vi "DetectCollisionImproved.vi"(0 "ball":dbl[](array[numeric]), 4 "Goal":dbl[](array[numeric]), 5 "our_robots":T1[](array[typedef]), 6 "Initial State":dbl[](array[numeric]), 7 "enemy_robots":T1[](array[typedef]), 8 "Is not first robot?":bool, 9 "element being analyzed":dbl[](array[numeric]), 10 "element already in path":dbl[](array[numeric]), 11 "Robot in":T1) -> (2 "Is there colision?":bool)   [LabVIEW 2017]
uses:
  Core/AI Robot.ctl
  Intel/Functions Enum.ctl
  Intel/AttackerStates.ctl
  PathDests.ctl
  PathDest.ctl
  <vilib>/Analysis/_algsub.llb/Real Vector Norm.vi
  <vilib>/Analysis/baseanly.llb/Real Dot Product.vi
  <vilib>/Analysis/NI_AALBase.lvlib
  <vilib>/Analysis/NI_AALPro.lvlib
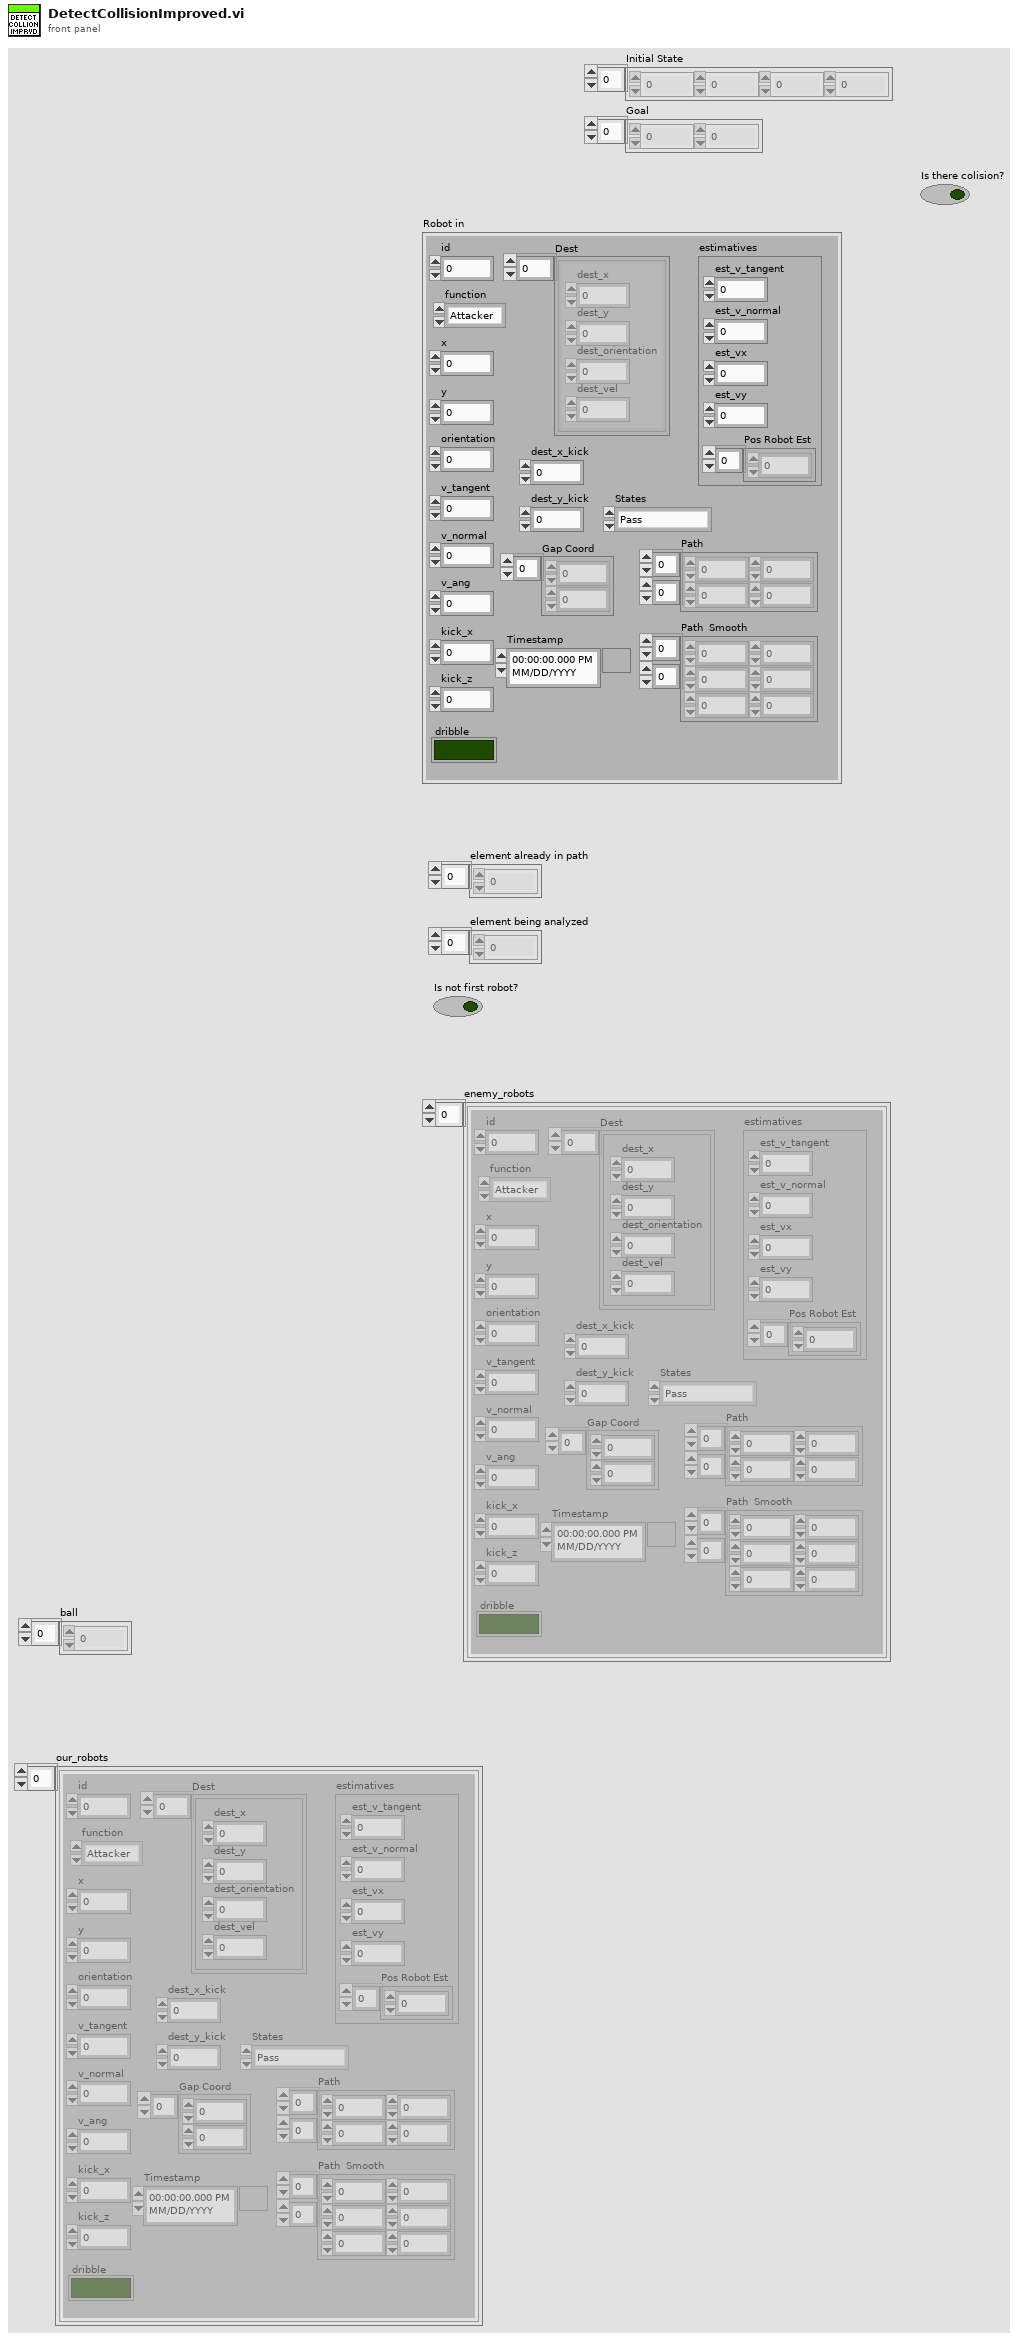
[diagram p1: front panel]
types:
  T1 = typedef "AI Robot.ctl" = cluster{"id":u32, "function":T2, "x":dbl, "y":dbl, "orientation":dbl, "v_tangent":dbl, "v_normal":dbl, "v_ang":dbl, "kick_x":dbl, "kick_z":dbl, "dribble":bool, "Timestamp":timestamp, "estimatives":cluster{"est_v_tangent":dbl, "est_v_normal":dbl, "est_vx":dbl, "est_vy":dbl, "Pos Robot Est":dbl[]}, "dest_x_kick":dbl, "dest_y_kick":dbl, "Gap Coord":dbl[], "States":T3, "Path ":dbl[][], "Path  Smooth":dbl[][], "Dest":T4}
  T2 = typedef "Functions Enum.ctl" = enum16{"Attacker", "Goalie", "Defender", "Striker", "Goto 0", "Dummy", "Kicker", "ZigZag"}
  T3 = typedef "AttackerStates.ctl" = enum16{"Pass", "GoToTangent", "BallGetting", "GoToKick", ""}
  T4 = typedef "PathDests.ctl" = T5[]
  T5 = typedef "PathDest.ctl" = cluster{"dest_x":dbl, "dest_y":dbl, "dest_orientation":dbl, "dest_vel":dbl}
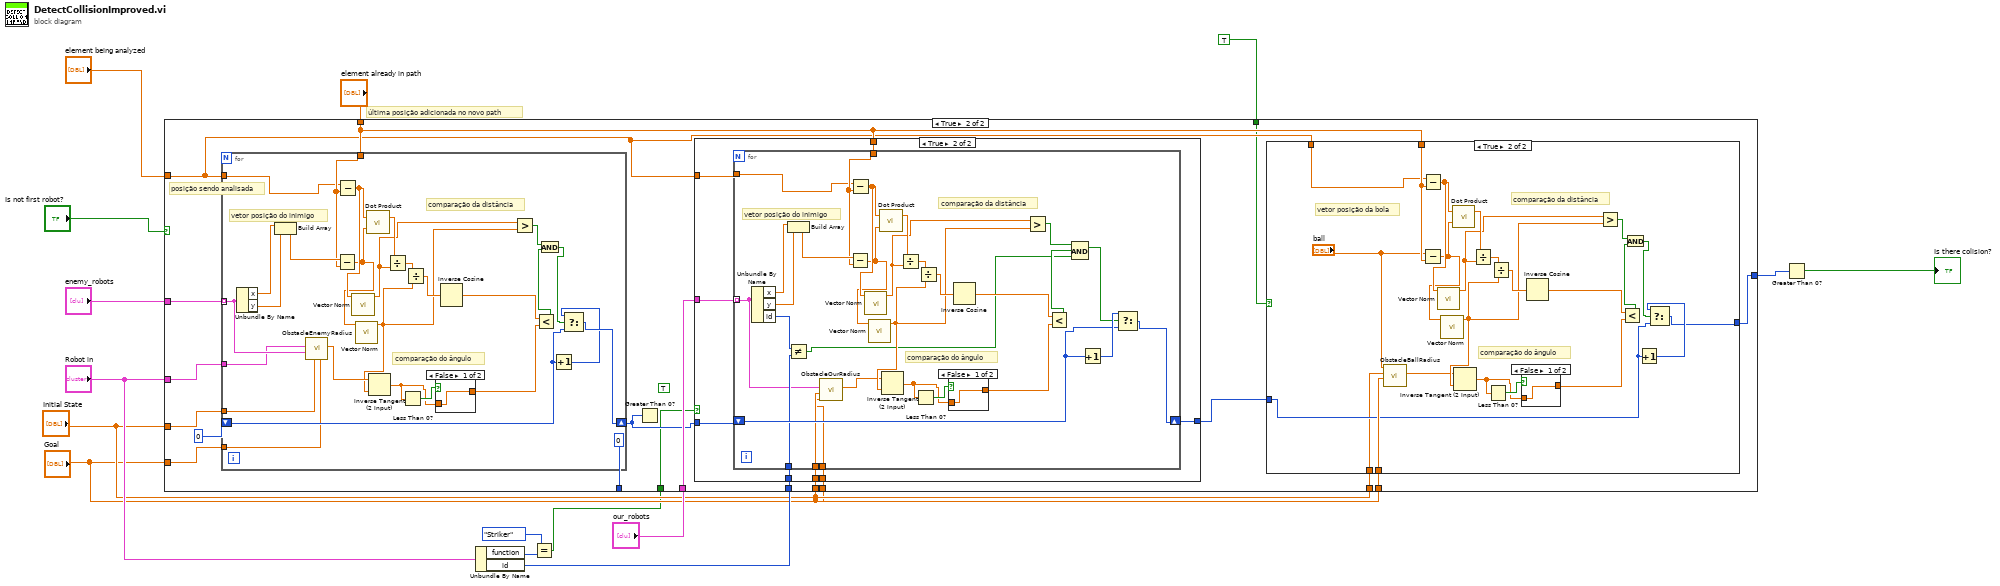
[diagram p0: block diagram]
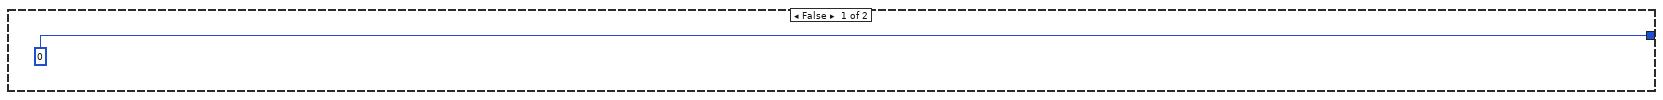
[diagram p2: hidden frame]
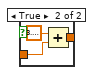
[diagram p4: hidden frame]
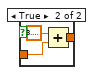
[diagram p6: hidden frame]
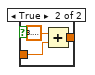
[diagram p7: hidden frame]
diagram:
  # "última posição adicionada no novo path"
  n1 = Unbundle By Name("Robot in") -> ("function"=w3:T2, "id"=w7:u32)
  n2 = Equal?(x=Functions_Enum."Striker", y=w3) -> (x = y?=w1:bool)
  n3 = case shown="True" "Is not first robot?" {
    tunnel: "enemy_robots" -> [_ w35]
    tunnel: "element being analyzed" -> [_ w23]
    tunnel: "element already in path" -> [_ w24]
    tunnel: [0 w20] -> w15
    tunnel: "Robot in" -> [_ w33]
    tunnel: "Initial State" -> [_ w32]
    tunnel: "Goal" -> [_ w31]
    tunnel: 0 -> [_ _]
    tunnel: "our_robots" -> [_ w30]
    tunnel: w7 -> [_ w29]
    tunnel: "Initial State" -> [_ w27]
    tunnel: "Goal" -> [_ w26]
    tunnel: "Initial State" -> [_ w22]
    tunnel: "Goal" -> [_ w21]
    tunnel: TRUE -> [_ w19]
    tunnel: w1 -> [_ w18]
    frame False {
    }
    frame True {
      (unwired) TRUE
      # "posição sendo analisada"
      n4 = for {
        tunnel: w35 -> [w111] mode=indexing
        shift-right: [w121] -> w28
        shift-left: 0 -> [w119]
        tunnel: w23 -> [w128]
        tunnel: w24 -> [w129]
        tunnel: w33 -> [w110]
        tunnel: w32 -> [w109]
        tunnel: w31 -> [w108]
        # "comparação do ângulo"
        # "comparação da distância"
        # "vetor posição do inimigo"
        n5 = Unbundle By Name(w111) -> ("x"=w132:dbl, "y"=w131:dbl)
        n6 = Build Array(w132, w131) -> (w130:dbl[])
        n7 = call "ObstacleEnemyRadius.vi"("Goal"=w108, "Initial State"=w109, "Robot enemy"=w111, "Robot in"=w110) -> ("obstacle enemy radius"=w107:dbl)  [unwired: 7 in]
        n8 = Subtract(x=w130, y=w129) -> (x-y=w122:dbl[])
        n9 = Subtract(x=w128, y=w129) -> (x-y=w126:dbl[])
        n10 = call-poly <vilib>:"Vector Norm.vi"("Input Vector"=w126) -> ("norm"=w118:dbl)  [unwired: 9 in, 1 out]
        n11 = call-poly <vilib>:"Vector Norm.vi"("Input Vector"=w122) -> ("norm"=w106:dbl)  [unwired: 9 in, 1 out]
        n12 = call-poly <vilib>:"Dot Product.vi"("Y Vector"=w122, "X Vector"=w126) -> ("X * Y"=w127:dbl)  [unwired: 1 out]
        n13 = Inverse Tangent (2 Input)(1:w106, 2:w107) -> (0:w113:dbl)
        n14 = Divide(x=w127, y=w118) -> (x/y=w125:dbl)
        n15 = Less Than 0?(x=w113) -> (x < 0?=w114:bool)
        n16 = Divide(x=w125, y=w106) -> (x/y=w124:dbl)
        n17 = case shown="False" w114 {
          tunnel: w113 -> [w133 w135]
          tunnel: [w133 w134] -> w112
          frame False {
          }
          frame True {
            n18 = Add(x=3.141592653589793, y=w135) -> (x+y=w134:dbl)
          }
        }
        n19 = Inverse Cosine(1:w124) -> (0:w123:dbl)
        n20 = Greater?(x=w118, y=w106) -> (0:w117:bool)
        n21 = Less?(x=w123, y=w112) -> (x < y?=w116:bool)
        n22 = And(x=w117, y=w116) -> (x .and. y?=w115:bool)
        n23 = Increment(x=w119) -> (x+1=w120:i32)
        n24 = Select(t=w120, s=w115, f=w119) -> (s? t:f=w121:i32)
      }
      n25 = Greater Than 0?(x=w28) -> ()  [unwired: 1 out]
      n26 = case shown="True" w18 {
        tunnel: w28 -> [w64 w72]
        tunnel: w30 -> [_ w71]
        tunnel: w24 -> [_ w70]
        tunnel: w23 -> [_ w69]
        tunnel: w29 -> [_ w68]
        tunnel: [w64 w67] -> w25
        tunnel: w27 -> [_ w66]
        tunnel: w26 -> [_ w65]
        frame False {
        }
        frame True {
          n27 = for {
            tunnel: w71 -> [w75] mode=indexing
            shift-right: [w90] -> w67
            shift-left: w72 -> [w81]
            tunnel: w69 -> [w97]
            tunnel: w70 -> [w98]
            tunnel: w68 -> [w78]
            tunnel: w66 -> [w74]
            tunnel: w65 -> [w73]
            # "comparação do ângulo"
            # "comparação da distância"
            # "vetor posição do inimigo"
            n28 = Unbundle By Name(w75) -> ("x"=w101:dbl, "y"=w100:dbl, "id"=w79:u32)
            n29 = Build Array(w101, w100) -> (w99:dbl[])
            n30 = Not Equal?(x=w79, y=w78) -> (x != y?=w77:bool)
            n31 = call "ObstacleOurRadius.vi"("Goal"=w73, "Initial State"=w74, "other robot"=w75) -> ("obstacle enemy radius"=w76:dbl)  [unwired: 8 in]
            n32 = Subtract(x=w99, y=w98) -> (x-y=w91:dbl[])
            n33 = Subtract(x=w97, y=w98) -> (x-y=w95:dbl[])
            n34 = call-poly <vilib>:"Vector Norm.vi"("Input Vector"=w95) -> ("norm"=w88:dbl)  [unwired: 9 in, 1 out]
            n35 = call-poly <vilib>:"Vector Norm.vi"("Input Vector"=w91) -> ("norm"=w82:dbl)  [unwired: 9 in, 1 out]
            n36 = call-poly <vilib>:"Dot Product.vi"("Y Vector"=w91, "X Vector"=w95) -> ("X * Y"=w96:dbl)  [unwired: 1 out]
            n37 = Inverse Tangent (2 Input)(1:w82, 2:w76) -> (0:w84:dbl)
            n38 = Divide(x=w96, y=w88) -> (x/y=w94:dbl)
            n39 = Less Than 0?(x=w84) -> (x < 0?=w85:bool)
            n40 = Divide(x=w94, y=w82) -> (x/y=w93:dbl)
            n41 = case shown="False" w85 {
              tunnel: w84 -> [w102 w104]
              tunnel: [w102 w103] -> w83
              frame False {
              }
              frame True {
                n42 = Add(x=3.141592653589793, y=w104) -> (x+y=w103:dbl)
              }
            }
            n43 = Inverse Cosine(1:w93) -> (0:w92:dbl)
            n44 = Greater?(x=w88, y=w82) -> (0:w87:bool)
            n45 = Less?(x=w92, y=w83) -> (x < y?=w86:bool)
            n46 = Compound Arithmetic op=AND(w87, w86, w77) -> (w80:bool)
            n47 = Increment(x=w81) -> (x+1=w89:i32)
            n48 = Select(t=w89, s=w80, f=w81) -> (s? t:f=w90:i32)
          }
        }
      }
      n49 = case shown="True" w19 {
        tunnel: w25 -> [w36 w39]
        tunnel: w24 -> [_ w44]
        tunnel: w23 -> [_ w43]
        tunnel: w22 -> [_ w37]
        tunnel: w21 -> [_ w40]
        tunnel: [w36 w38] -> w20
        frame False {
        }
        frame True {
          # "comparação do ângulo"
          # "comparação da distância"
          # "vetor posição da bola"
          n50 = call "ObstacleBallRadius.vi"("Goal"=w40, "Initial State"=w37, "ball"="ball") -> ("obstacle enemy radius"=w42:dbl)  [unwired: 8 in]
          n51 = Subtract(x="ball", y=w44) -> (x-y=w54:dbl[])
          n52 = Subtract(x=w43, y=w44) -> (x-y=w58:dbl[])
          n53 = call-poly <vilib>:"Vector Norm.vi"("Input Vector"=w58) -> ("norm"=w52:dbl)  [unwired: 9 in, 1 out]
          n54 = call-poly <vilib>:"Vector Norm.vi"("Input Vector"=w54) -> ("norm"=w45:dbl)  [unwired: 9 in, 1 out]
          n55 = call-poly <vilib>:"Dot Product.vi"("Y Vector"=w54, "X Vector"=w58) -> ("X * Y"=w59:dbl)  [unwired: 1 out]
          n56 = Inverse Tangent (2 Input)(1:w45, 2:w42) -> (0:w47:dbl)
          n57 = Divide(x=w59, y=w52) -> (x/y=w57:dbl)
          n58 = Less Than 0?(x=w47) -> (x < 0?=w48:bool)
          n59 = Divide(x=w57, y=w45) -> (x/y=w56:dbl)
          n60 = case shown="False" w48 {
            tunnel: w47 -> [w60 w62]
            tunnel: [w60 w61] -> w46
            frame False {
            }
            frame True {
              n61 = Add(x=3.141592653589793, y=w62) -> (x+y=w61:dbl)
            }
          }
          n62 = Inverse Cosine(1:w56) -> (0:w55:dbl)
          n63 = Greater?(x=w52, y=w45) -> (0:w51:bool)
          n64 = Less?(x=w55, y=w46) -> (x < y?=w50:bool)
          n65 = And(x=w51, y=w50) -> (x .and. y?=w49:bool)
          n66 = Increment(x=w39) -> (x+1=w53:i32)
          n67 = Select(t=w53, s=w49, f=w39) -> (s? t:f=w38:i32)
        }
      }
    }
  }
  n68 = Greater Than 0?(x=w15) -> (x > 0?=→"Is there colision?":bool)
